vi "Accurate Measure_BU.vi"(0 "DMM ref":refnum<visa-resource-name>, 1 "channel_count":i32=11, 2 "P_current_count":i32, 3 "N_current_count":i32, 5 "DMM error":errorcluster, 7 "Enable DMM-\nRelay":bool=TRUE, 9 "ESP32 ref":refnum<visa-resource-name>, 11 "ESP32 error":errorcluster, 12 "current_mode":u8[](array[numeric])=[0, 0, 0, 0, 0, 0, 0, 0, 0, 0, 0]) -> ()   [LabVIEW 2023]
uses:
  <instrlib>/Agilent 3446X Series/Agilent 3446X Series.lvlib
panel:
  out "time_out_count":i32
  in  "Timeout":i32=100
  out "Arithmetic Mean 3":dbl[](array[numeric])
  out "+ STD":dbl[](array[numeric])
  out "Arithmetic Mean 2":dbl[](array[numeric])
  out "-STD":dbl[](array[numeric])
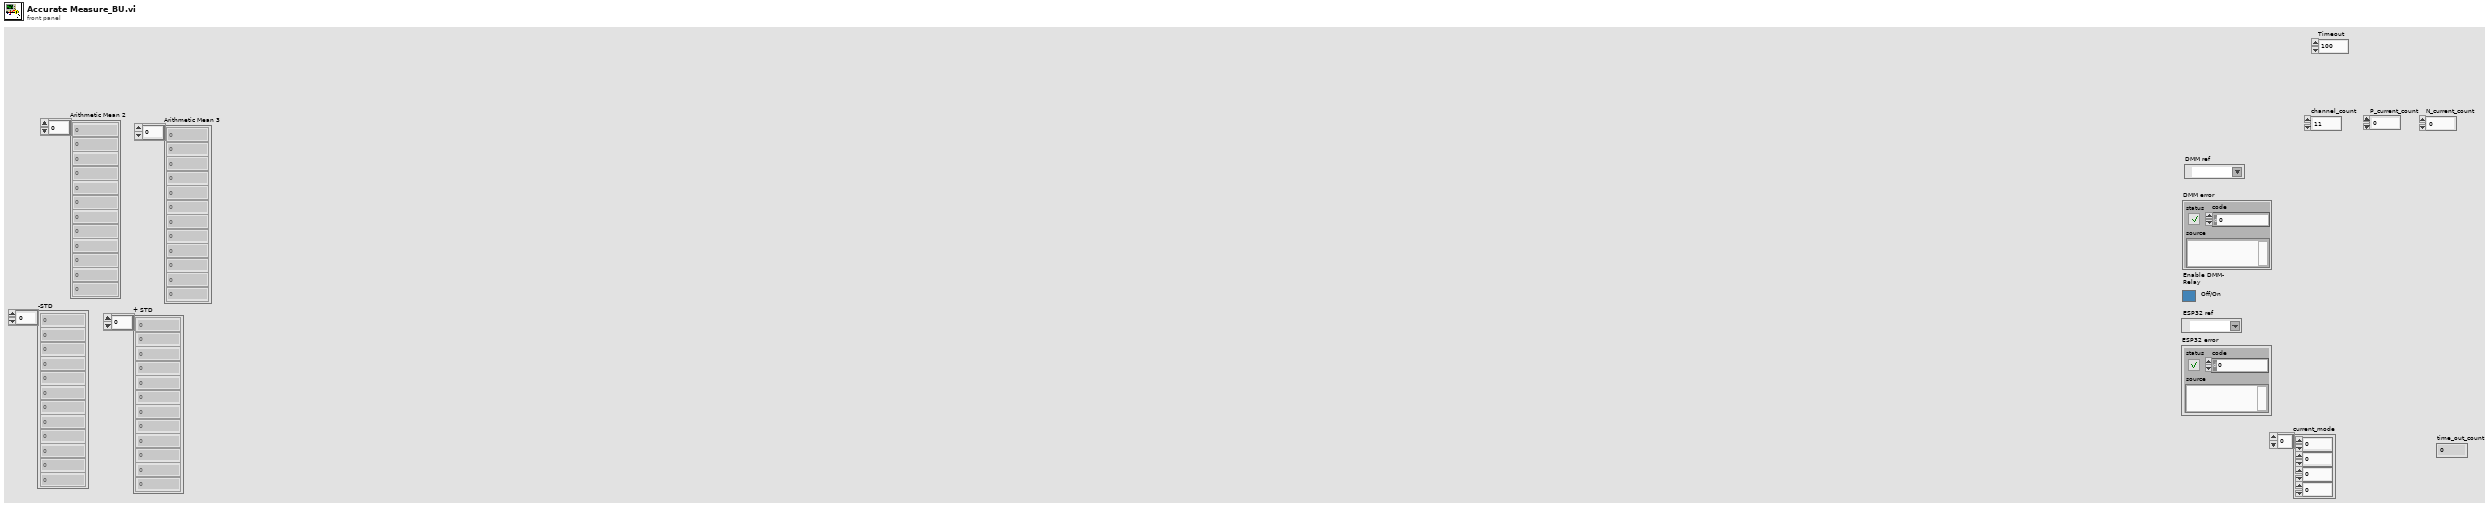
[diagram p1: front panel]
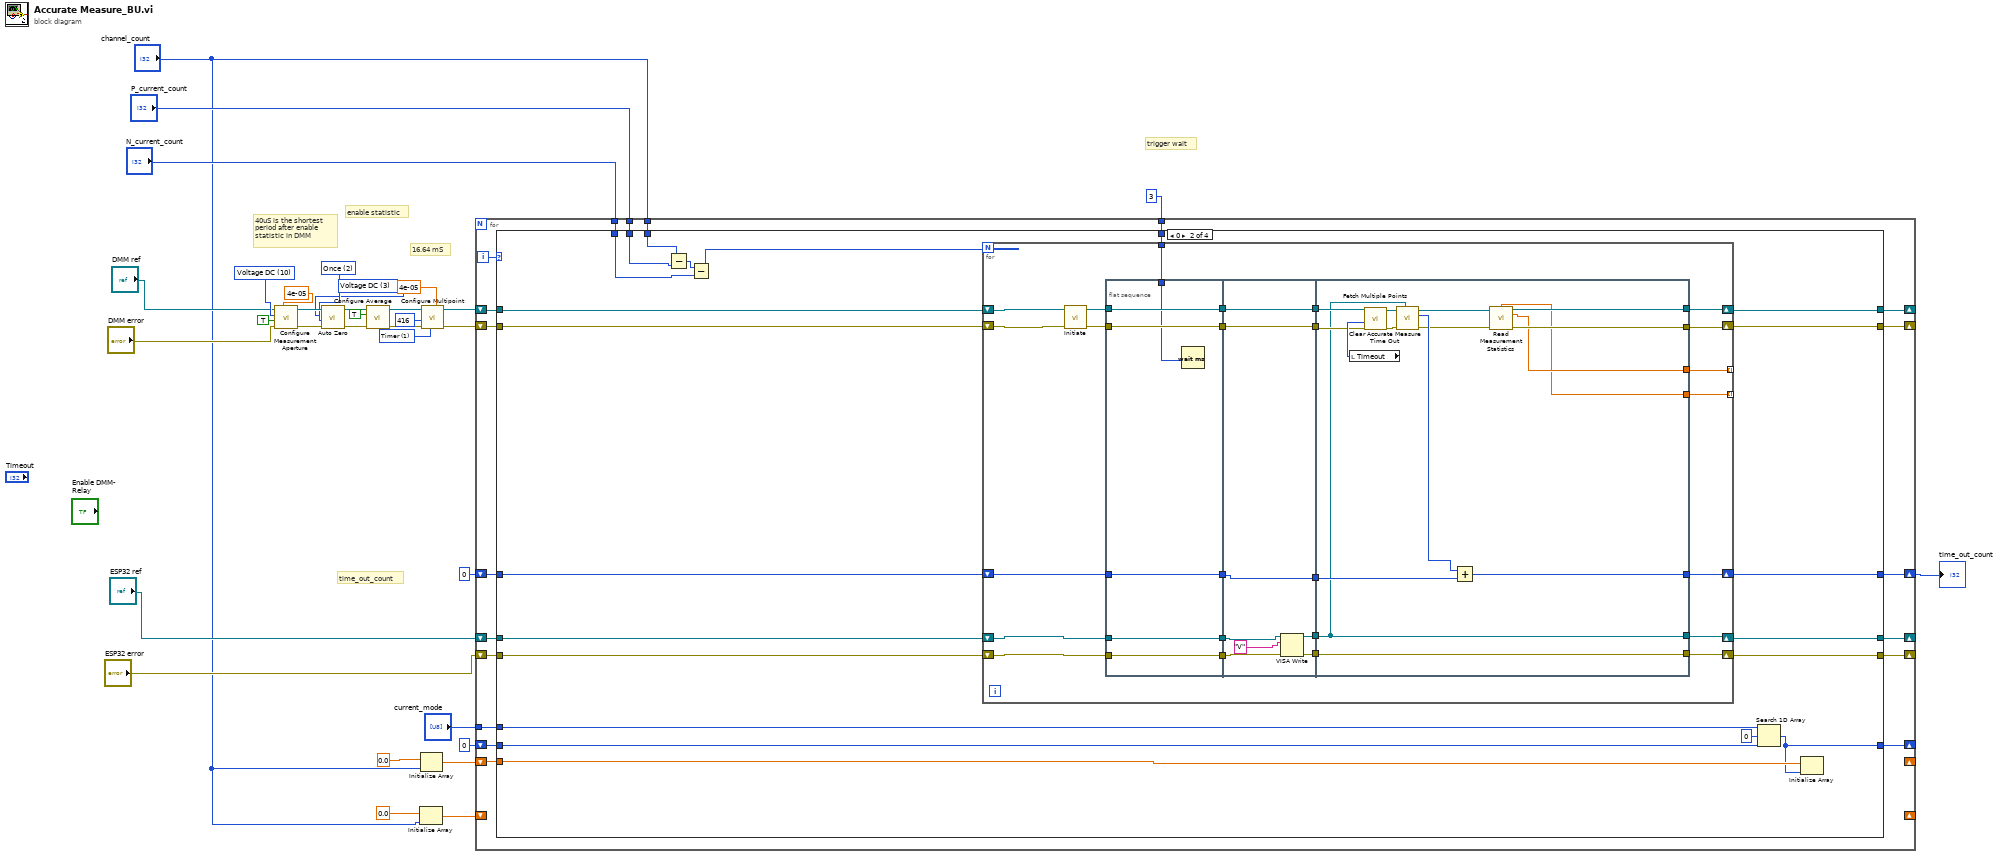
[diagram p0: block diagram]
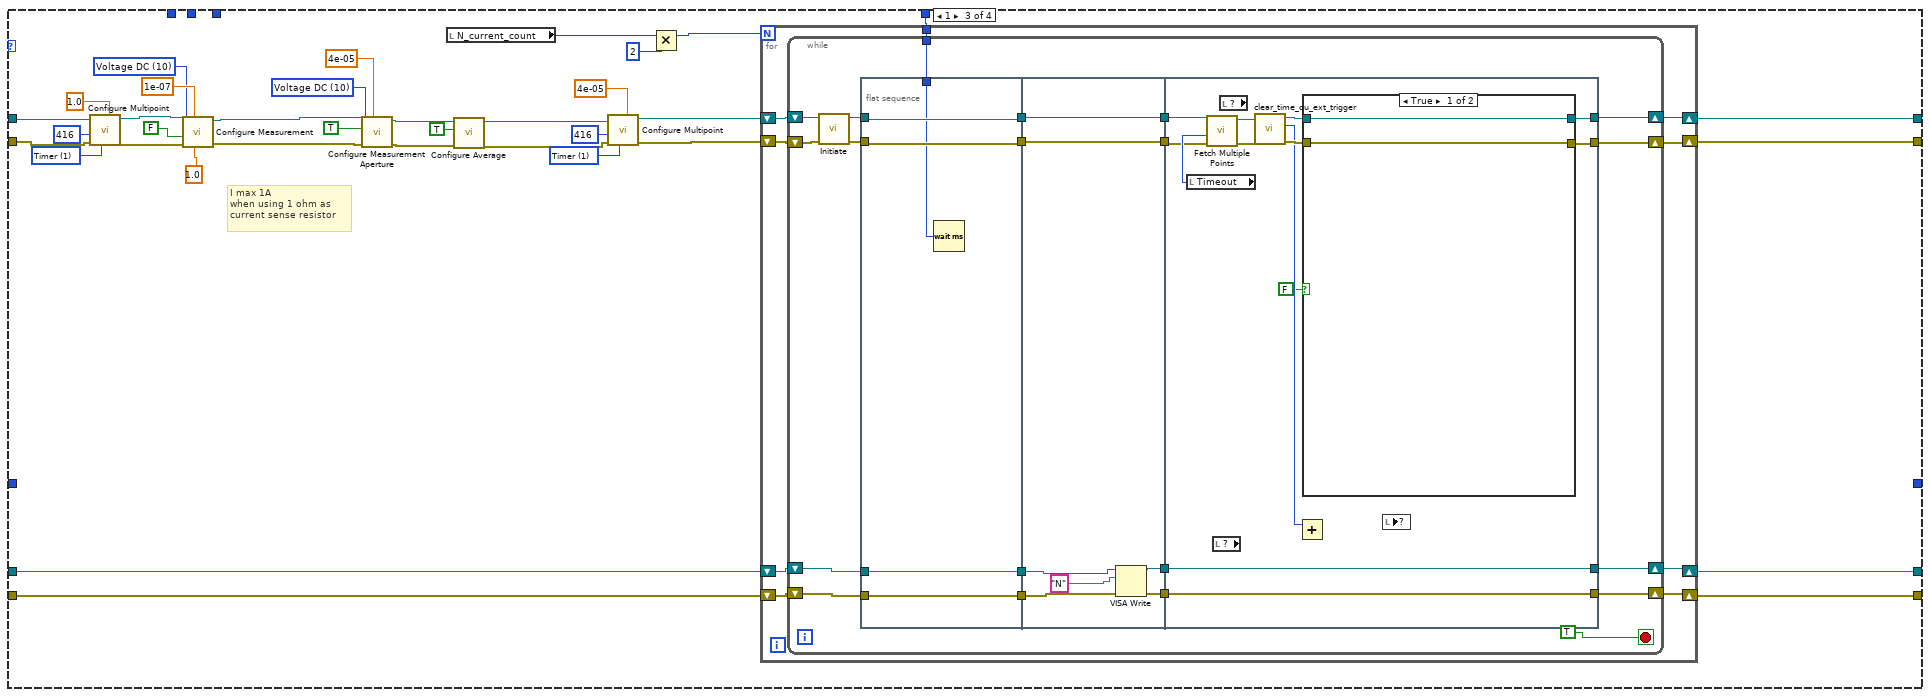
[diagram p3: hidden frame]
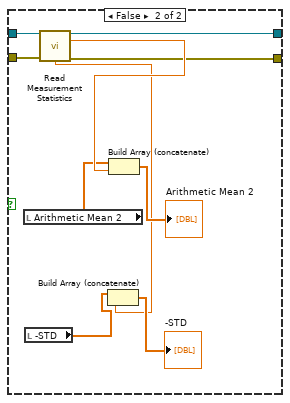
[diagram p4: hidden frame]
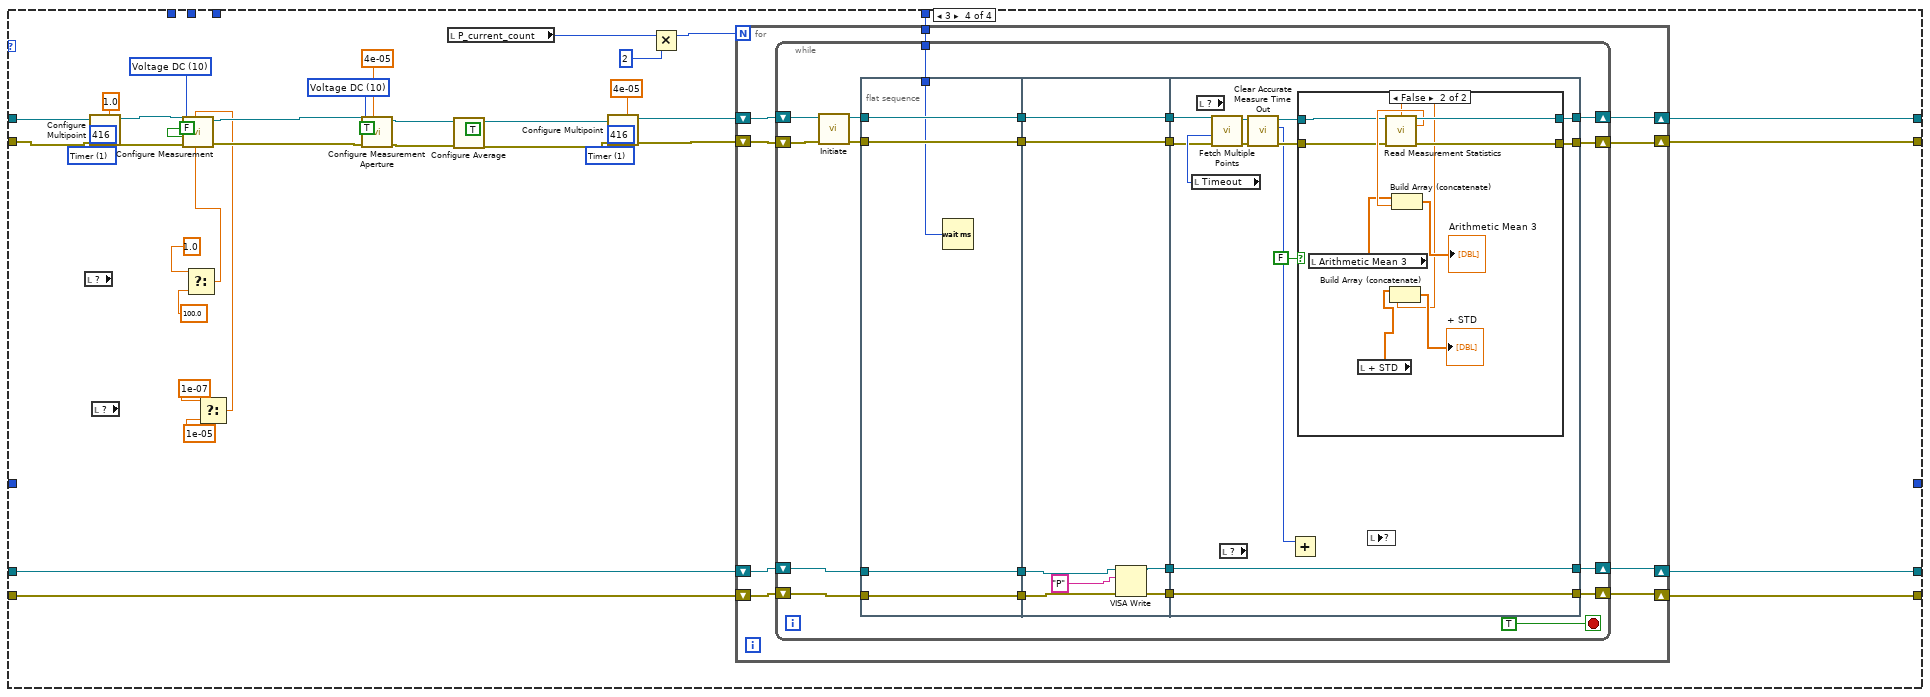
[diagram p5: hidden frame]
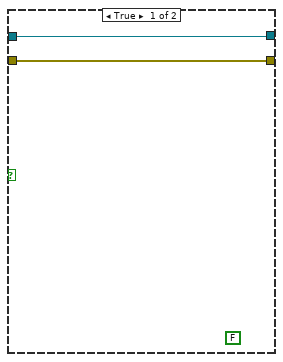
[diagram p6: hidden frame]
diagram:
  w20 = 1 items=["Immediate", "Timer"] ("Sample Source (0: Immediate)")
  w27 = 3 items=["Current DC", "Resistance", "Temperature", "Voltage DC"] ("Zero Type (0: Current DC)")
  w28 = 2 items=["Disable", "Enable", "Once"] ("Auto Zero (1: Enable)")
  w24 = 10 items=["Continuity", "Current AC", "Current DC", "Diode", "Frequency", "Resistance 4-wire", "Period", "Resistance 2-wire", "Temperature", "Voltage AC", "Voltage DC", "Voltage DC Ratio", "Capacitance"] ("Measurement Function (0: Continuity)")
  # "time_out_count"
  # "trigger wait"
  # "16.64 mS"
  # "enable statistic"
  # "40uS is the shortest\nperiod after enable \nstatistic in DMM"
  n1 = call <instrlib>:"Configure Measurement Aperture.vi"("Aperture Time (0.1s)"=4e-05, "error in (no error)"="DMM error", "Enable Aperture (F: Disable)"=TRUE, "Measurement Function (0: Continuity)"=w24, "VISA resource name"="DMM ref") -> ("error out"=w31:errorcluster, "VISA resource name out"=w30:refnum<visa-resource-name>)  [unwired: 5 in]
  n2 = call <instrlib>:"Auto Zero.vi"("error in (no error)"=w31, "Auto Zero (1: Enable)"=w28, "Zero Type (0: Current DC)"=w27, "VISA resource name"=w30) -> ("error out"=w33:errorcluster, "VISA resource name out"=w32:refnum<visa-resource-name>)  [unwired: 6 in]
  n3 = call <instrlib>:"Configure Average.vi"("error in (no error)"=w33, "Enable Statistics (F: Disable)"=TRUE, "VISA resource name"=w32) -> ("error out"=w22:errorcluster, "VISA resource name out"=w23:refnum<visa-resource-name>)  [unwired: 7 in]
  n4 = Initialize Array(0.0 ("Arithmetic Mean"), "channel_count") -> (w2:dbl[])
  n5 = Initialize Array(0.0 ("Arithmetic Mean"), "channel_count") -> (w3:dbl[])
  n6 = call <instrlib>:"Configure Multipoint.vi"("Sample Interval (1 Second)"=4e-05, "Sample Source (0: Immediate)"=w20, "error in (no error)"=w22, "Sample Count (1)"=416, "VISA resource name"=w23) -> ("error out"=w17:errorcluster, "VISA resource name out"=w18:refnum<visa-resource-name>)  [unwired: 2 in, 3 out]
  n7 = for {
    shift-right: [w50] -> _
    shift-left: "ESP32 ref" -> [w52]
    shift-right: [w49] -> _
    shift-left: "ESP32 error" -> [w51]
    shift-right: [w46] -> _
    shift-left: w18 -> [w48]
    shift-right: [w45] -> _
    shift-left: w17 -> [w47]
    tunnel: "channel_count" -> [w44]
    tunnel: "P_current_count" -> [w43]
    tunnel: "N_current_count" -> [w42]
    tunnel: u32 3 ("milliseconds to wait") -> [w41]
    shift-right: [w40] -> w8
    shift-left: 0 -> [w39]
    tunnel: "current_mode" -> [w38]
    shift-right: _ -> [_]
    shift-left: w3 -> [w34]
    shift-right: _ -> [_]
    shift-left: w2 -> [_]
    shift-right: [w36] -> _
    shift-left: 0 ("index of element") -> [w35]
    i -> [w37]
    n8 = case shown="0" w37 {
      tunnel: w52 -> [w54 w73 w168 w274]
      tunnel: w51 -> [w53 w72 w167 w273]
      tunnel: [w54 w69 w164 w270] -> w50
      tunnel: [w53 w68 w163 w269] -> w49
      tunnel: w48 -> [w56 w75 w154 w262]
      tunnel: w47 -> [w55 w74 w153 w261]
      tunnel: [w56 w71 w166 w272] -> w46
      tunnel: [w55 w70 w165 w271] -> w45
      tunnel: w44 -> [_ w67 _ _]
      tunnel: w43 -> [_ w66 _ _]
      tunnel: w42 -> [_ w65 _ _]
      tunnel: [_ w63 _ _] -> w40
      tunnel: w41 -> [_ w64 w133 w235]
      tunnel: w39 -> [_ w62 _ _]
      tunnel: w38 -> [_ w61 _ _]
      tunnel: [_ w57 _ _] -> w36
      tunnel: w35 -> [_ w59 _ _]
      tunnel: w34 -> [_ w58 _ _]
      frame Default {
      }
      frame 0 {
        n9 = Subtract(x=w67, y=w66) -> (x-y=w77:i32)
        n10 = Subtract(x=w77, y=w65) -> (x-y=w76:i32)
        n11 = for {
          N: w76 -> [_]
          shift-right: [w98] -> w71
          shift-left: w75 -> [w102]
          shift-right: [w97] -> w70
          shift-left: w74 -> [w101]
          shift-right: [w96] -> w69
          shift-left: w73 -> [w100]
          shift-right: [w95] -> w68
          shift-left: w72 -> [w99]
          tunnel: w64 -> [w81]
          shift-right: [w80] -> w63
          shift-left: w62 -> [w94]
          tunnel: [w79] -> _ mode=indexing
          tunnel: [w78] -> _ mode=indexing
          n12 = call <instrlib>:"Initiate.vi"("error in (no error)"=w101, "VISA resource name"=w102) -> ("error out"=w82:errorcluster, "VISA resource name out"=w83:refnum<visa-resource-name>)  [unwired: 8 in]
          n13 = flat-sequence {
            tunnel: [w108] -> w93
            tunnel: w100 -> [w108]
            tunnel: [w107] -> w92
            tunnel: w99 -> [w107]
            tunnel: w83 -> [w106]
            tunnel: [w106] -> w91
            tunnel: [w105] -> w90
            tunnel: w82 -> [w105]
            tunnel: [w104] -> w89
            tunnel: w94 -> [w104]
            tunnel: w81 -> [w103]
            tunnel: w93 -> [w116]
            tunnel: w92 -> [w115]
            tunnel: w91 -> [w114]
            tunnel: [w114] -> w85
            tunnel: w90 -> [w113]
            tunnel: [w113] -> w86
            tunnel: [w112] -> w87
            tunnel: [w111] -> w88
            tunnel: w89 -> [w109]
            tunnel: [w109] -> w84
            tunnel: [w132] -> w95
            tunnel: [w119] -> w96
            tunnel: [w123] -> w97
            tunnel: [w124] -> w98
            tunnel: w88 -> [w132]
            tunnel: w87 -> [w119]
            tunnel: w86 -> [w130]
            tunnel: w85 -> [w129]
            tunnel: [w125] -> w80
            tunnel: w84 -> [w120]
            tunnel: [w118] -> w79
            tunnel: [w117] -> w78
            frame #0 {
              n14 = Wait (ms)(milliseconds to wait=w103) -> ()  [unwired: 1 out]
            }
            frame #1 {
              n15 = VISA Write(VISA resource name=w116, write buffer="V" ("data in"), error in (no error)=w115) -> (VISA resource name out=w112:refnum<visa-resource-name>, error out=w111:errorcluster)  [unwired: 1 out]
            }
            frame #2 {
              n16 = local read "Timeout"() -> (w131:i32)
              n17 = call <instrlib>:"Fetch Multiple Points.vi"("error in (no error)"=w130, "Timeout (10000 ms)"=w131, "VISA resource name"=w129) -> ("error out"=w127:errorcluster, "VISA resource name out"=w128:refnum<visa-resource-name>)  [unwired: 1 in, 6 out]
              n18 = call "Clear Accurate Measure Time Out.vi"("ESP32 ref"=w119, "error in (no error)"=w127, "DMM ref"=w128) -> ("error out"=w121:errorcluster, "Time out count"=w126:i32, "VISA Refnum out"=w122:refnum<visa-resource-name>)  [unwired: 5 in, 1 out]
              n19 = Add(x=w126, y=w120) -> (x+y=w125:i32)
              n20 = call <instrlib>:"Read Measurement Statistics.vi"("VISA resource name"=w122, "error in (no error)"=w121) -> ("Standard Deviation"=w117:dbl, "VISA resource name out"=w124:refnum<visa-resource-name>, "Arithmetic Mean"=w118:dbl, "error out"=w123:errorcluster)  [unwired: 6 in, 4 out]
            }
          }
        }
        n21 = Search 1D Array(1D array=w61, element=u8 0, start index (0)=w59) -> (index of element=w57:i32)
        n22 = Initialize Array(w58, w57) -> ()  [unwired: 1 out]
      }
      frame 1 {
        w146 = 1 items=["Immediate", "Timer"] ("Sample Source (0: Immediate)")
        w149 = 10 items=["Continuity", "Current AC", "Current DC", "Diode", "Frequency", "Resistance 4-wire", "Period", "Resistance 2-wire", "Temperature", "Voltage AC", "Voltage DC", "Voltage DC Ratio", "Capacitance"] ("Measurement Function (0: Continuity)")
        w156 = 1 items=["Immediate", "Timer"] ("Sample Source (0: Immediate)")
        w158 = 10 items=["Continuity", "Current AC", "Current DC", "Diode", "Frequency", "Resistance 4-wire", "Period", "Resistance 2-wire", "Temperature", "Voltage AC", "Voltage DC", "Voltage DC Ratio", "Capacitance"] ("Measurement Function (10: Voltage DC)")
        # "I max 1A\nwhen using 1 ohm as \ncurrent sense resistor"
        n23 = call <instrlib>:"Configure Multipoint.vi"("Sample Interval (1 Second)"=1.0, "Sample Source (0: Immediate)"=w156, "error in (no error)"=w153, "Sample Count (1)"=416, "VISA resource name"=w154) -> ("error out"=w138:errorcluster, "VISA resource name out"=w137:refnum<visa-resource-name>)  [unwired: 2 in, 3 out]
        n24 = call <instrlib>:"Configure Measurement.vi"("Manual Range (1)"=1.0, "Absolute Resolution (1E-6)"=1e-07, "error in (no error)"=w138, "Auto Range (T: Enable)"=FALSE, "Measurement Function (10: Voltage DC)"=w158, "VISA resource name"=w137) -> ("error out"=w135:errorcluster, "VISA resource name out"=w136:refnum<visa-resource-name>)  [unwired: 4 out]
        n25 = call <instrlib>:"Configure Measurement Aperture.vi"("Aperture Time (0.1s)"=4e-05, "error in (no error)"=w135, "Enable Aperture (F: Disable)"=TRUE, "Measurement Function (0: Continuity)"=w149, "VISA resource name"=w136) -> ("error out"=w140:errorcluster, "VISA resource name out"=w141:refnum<visa-resource-name>)  [unwired: 5 in]
        n26 = local read "N_current_count"() -> (w162:i32)
        n27 = call <instrlib>:"Configure Average.vi"("error in (no error)"=w140, "Enable Statistics (F: Disable)"=TRUE, "VISA resource name"=w141) -> ("error out"=w139:errorcluster, "VISA resource name out"=w134:refnum<visa-resource-name>)  [unwired: 7 in]
        n28 = call <instrlib>:"Configure Multipoint.vi"("Sample Interval (1 Second)"=4e-05, "Sample Source (0: Immediate)"=w146, "error in (no error)"=w139, "Sample Count (1)"=416, "VISA resource name"=w134) -> ("error out"=w143:errorcluster, "VISA resource name out"=w144:refnum<visa-resource-name>)  [unwired: 2 in, 3 out]
        n29 = Multiply(x=w162, y=2) -> (x*y=w152:i32)
        n30 = for {
          N: w152 -> [_]
          shift-right: [w173] -> w166
          shift-left: w144 -> [w177]
          shift-right: [w172] -> w165
          shift-left: w143 -> [w176]
          shift-right: [w171] -> w164
          shift-left: w168 -> [w175]
          shift-right: [w170] -> w163
          shift-left: w167 -> [w174]
          tunnel: w133 -> [w169]
          n31 = while {
            shift-right: [w183] -> w173
            shift-left: w177 -> [w189]
            shift-right: [w182] -> w172
            shift-left: w176 -> [w188]
            shift-right: [w181] -> w171
            shift-left: w175 -> [w187]
            shift-right: [w180] -> w170
            shift-left: w174 -> [w186]
            tunnel: w169 -> [w178]
            stop <- TRUE stop-if-true
            n32 = call <instrlib>:"Initiate.vi"("error in (no error)"=w188, "VISA resource name"=w189) -> ("error out"=w184:errorcluster, "VISA resource name out"=w185:refnum<visa-resource-name>)  [unwired: 8 in]
            n33 = flat-sequence {
              tunnel: [w202] -> w197
              tunnel: w187 -> [w202]
              tunnel: [w201] -> w196
              tunnel: w186 -> [w201]
              tunnel: w185 -> [w200]
              tunnel: [w200] -> w195
              tunnel: [w199] -> w194
              tunnel: w184 -> [w199]
              tunnel: w178 -> [w198]
              tunnel: w197 -> [w209]
              tunnel: w196 -> [w208]
              tunnel: w195 -> [w207]
              tunnel: [w207] -> w193
              tunnel: w194 -> [w206]
              tunnel: [w206] -> w192
              tunnel: [w205] -> w191
              tunnel: [w204] -> w190
              tunnel: w193 -> [w218]
              tunnel: w192 -> [w219]
              tunnel: [w213] -> w183
              tunnel: [w212] -> w182
              tunnel: [w222] -> w181
              tunnel: w191 -> [w222]
              tunnel: [w221] -> w180
              tunnel: w190 -> [w221]
              frame #0 {
                n34 = Wait (ms)(milliseconds to wait=w198) -> ()  [unwired: 1 out]
              }
              frame #1 {
                n35 = VISA Write(VISA resource name=w209, write buffer="N" ("data in"), error in (no error)=w208) -> (VISA resource name out=w205:refnum<visa-resource-name>, error out=w204:errorcluster)  [unwired: 1 out]
              }
              frame #2 {
                n36 = local read "Timeout"() -> (w220:i32)
                n37 = call <instrlib>:"Fetch Multiple Points.vi"("error in (no error)"=w219, "Timeout (10000 ms)"=w220, "VISA resource name"=w218) -> ("error out"=w216:errorcluster, "VISA resource name out"=w217:refnum<visa-resource-name>)  [unwired: 1 in, 6 out]
                n38 = local read item#-1() -> ()  [unwired: 1 out]
                n39 = local read item#-1() -> ()  [unwired: 1 out]
                n40 = call "clear_time_ou_ext_trigger.vi"("error in (no error)"=w216, "VISA Refnum in"=w217) -> ("error out"=w214:errorcluster, "Time out count"=w211:i32, "VISA Refnum out"=w215:refnum<visa-resource-name>)  [unwired: 6 in, 1 out]
                n41 = Add(x=w211) -> ()  [unwired: 1 in, 1 out]
                n42 = case shown="True" FALSE {
                  tunnel: w215 -> [w224 w228]
                  tunnel: w214 -> [w223 w227]
                  tunnel: [w224 w226] -> w213
                  tunnel: [w223 w225] -> w212
                  frame True {
                  }
                  frame False {
                    n43 = local read "Arithmetic Mean 2"() -> (w233:dbl[])
                    n44 = local read "-STD"() -> (w231:dbl[])
                    n45 = call <instrlib>:"Read Measurement Statistics.vi"("VISA resource name"=w228, "error in (no error)"=w227) -> ("Standard Deviation"=w229:dbl, "VISA resource name out"=w226:refnum<visa-resource-name>, "Arithmetic Mean"=w234:dbl, "error out"=w225:errorcluster)  [unwired: 6 in, 4 out]
                    n46 = Build Array (concatenate)(w231, w229) -> (→"-STD":dbl[])
                    n47 = Build Array (concatenate)(w233, w234) -> (→"Arithmetic Mean 2":dbl[])
                  }
                }
                n48 = local read item#-1() -> ()  [unwired: 1 in]
              }
            }
          }
        }
      }
      frame 3 {
        w254 = 1 items=["Immediate", "Timer"] ("Sample Source (0: Immediate)")
        w257 = 10 items=["Continuity", "Current AC", "Current DC", "Diode", "Frequency", "Resistance 4-wire", "Period", "Resistance 2-wire", "Temperature", "Voltage AC", "Voltage DC", "Voltage DC Ratio", "Capacitance"] ("Measurement Function (0: Continuity)")
        w264 = 1 items=["Immediate", "Timer"] ("Sample Source (0: Immediate)")
        w266 = 10 items=["Continuity", "Current AC", "Current DC", "Diode", "Frequency", "Resistance 4-wire", "Period", "Resistance 2-wire", "Temperature", "Voltage AC", "Voltage DC", "Voltage DC Ratio", "Capacitance"] ("Measurement Function (10: Voltage DC)")
        n49 = local read item#-1() -> ()  [unwired: 1 out]
        n50 = call <instrlib>:"Configure Multipoint.vi"("Sample Interval (1 Second)"=1.0, "Sample Source (0: Immediate)"=w264, "error in (no error)"=w261, "Sample Count (1)"=416, "VISA resource name"=w262) -> ("error out"=w246:errorcluster, "VISA resource name out"=w245:refnum<visa-resource-name>)  [unwired: 2 in, 3 out]
        n51 = local read item#-1() -> ()  [unwired: 1 out]
        n52 = Select(t=1.0 ("Manual Range (1)"), f=100.0 ("Manual Range (1)")) -> (s? t:f=w239:dbl)  [unwired: 1 in]
        n53 = Select(t=1e-07 ("Absolute Resolution (1E-6)"), f=1e-05 ("Absolute Resolution (1E-6)")) -> (s? t:f=w236:dbl)  [unwired: 1 in]
        n54 = call <instrlib>:"Configure Measurement.vi"("Manual Range (1)"=w239, "Absolute Resolution (1E-6)"=w236, "error in (no error)"=w246, "Auto Range (T: Enable)"=FALSE, "Measurement Function (10: Voltage DC)"=w266, "VISA resource name"=w245) -> ("error out"=w243:errorcluster, "VISA resource name out"=w244:refnum<visa-resource-name>)  [unwired: 4 out]
        n55 = call <instrlib>:"Configure Measurement Aperture.vi"("Aperture Time (0.1s)"=4e-05, "error in (no error)"=w243, "Enable Aperture (F: Disable)"=TRUE, "Measurement Function (0: Continuity)"=w257, "VISA resource name"=w244) -> ("error out"=w248:errorcluster, "VISA resource name out"=w249:refnum<visa-resource-name>)  [unwired: 5 in]
        n56 = local read "P_current_count"() -> (w268:i32)
        n57 = call <instrlib>:"Configure Average.vi"("error in (no error)"=w248, "Enable Statistics (F: Disable)"=TRUE, "VISA resource name"=w249) -> ("error out"=w247:errorcluster, "VISA resource name out"=w242:refnum<visa-resource-name>)  [unwired: 7 in]
        n58 = call <instrlib>:"Configure Multipoint.vi"("Sample Interval (1 Second)"=4e-05, "Sample Source (0: Immediate)"=w254, "error in (no error)"=w247, "Sample Count (1)"=416, "VISA resource name"=w242) -> ("error out"=w251:errorcluster, "VISA resource name out"=w252:refnum<visa-resource-name>)  [unwired: 2 in, 3 out]
        n59 = Multiply(x=w268, y=2) -> (x*y=w260:i32)
        n60 = for {
          N: w260 -> [_]
          shift-right: [w279] -> w272
          shift-left: w252 -> [w283]
          shift-right: [w278] -> w271
          shift-left: w251 -> [w282]
          shift-right: [w277] -> w270
          shift-left: w274 -> [w281]
          shift-right: [w276] -> w269
          shift-left: w273 -> [w280]
          tunnel: w235 -> [w275]
          n61 = while {
            shift-right: [w289] -> w279
            shift-left: w283 -> [w295]
            shift-right: [w288] -> w278
            shift-left: w282 -> [w294]
            shift-right: [w287] -> w277
            shift-left: w281 -> [w293]
            shift-right: [w286] -> w276
            shift-left: w280 -> [w292]
            tunnel: w275 -> [w284]
            stop <- TRUE stop-if-true
            n62 = call <instrlib>:"Initiate.vi"("error in (no error)"=w294, "VISA resource name"=w295) -> ("error out"=w290:errorcluster, "VISA resource name out"=w291:refnum<visa-resource-name>)  [unwired: 8 in]
            n63 = flat-sequence {
              tunnel: [w308] -> w303
              tunnel: w293 -> [w308]
              tunnel: [w307] -> w302
              tunnel: w292 -> [w307]
              tunnel: w291 -> [w306]
              tunnel: [w306] -> w301
              tunnel: [w305] -> w300
              tunnel: w290 -> [w305]
              tunnel: w284 -> [w304]
              tunnel: w303 -> [w315]
              tunnel: w302 -> [w314]
              tunnel: w301 -> [w313]
              tunnel: [w313] -> w299
              tunnel: w300 -> [w312]
              tunnel: [w312] -> w298
              tunnel: [w311] -> w297
              tunnel: [w310] -> w296
              tunnel: w299 -> [w322]
              tunnel: w298 -> [w323]
              tunnel: [w328] -> w289
              tunnel: [w327] -> w288
              tunnel: [w326] -> w287
              tunnel: w297 -> [w326]
              tunnel: [w325] -> w286
              tunnel: w296 -> [w325]
              frame #0 {
                n64 = Wait (ms)(milliseconds to wait=w304) -> ()  [unwired: 1 out]
              }
              frame #1 {
                n65 = VISA Write(VISA resource name=w315, write buffer="P" ("data in"), error in (no error)=w314) -> (VISA resource name out=w311:refnum<visa-resource-name>, error out=w310:errorcluster)  [unwired: 1 out]
              }
              frame #2 {
                n66 = local read "Timeout"() -> (w324:i32)
                n67 = local read item#-1() -> ()  [unwired: 1 out]
                n68 = call <instrlib>:"Fetch Multiple Points.vi"("error in (no error)"=w323, "Timeout (10000 ms)"=w324, "VISA resource name"=w322) -> ("error out"=w320:errorcluster, "VISA resource name out"=w321:refnum<visa-resource-name>)  [unwired: 1 in, 6 out]
                n69 = local read item#-1() -> ()  [unwired: 1 out]
                n70 = call "Clear Accurate Measure Time Out.vi"("error in (no error)"=w320, "DMM ref"=w321) -> ("error out"=w318:errorcluster, "Time out count"=w317:i32, "VISA Refnum out"=w319:refnum<visa-resource-name>)  [unwired: 6 in, 1 out]
                n71 = Add(x=w317) -> ()  [unwired: 1 in, 1 out]
                n72 = case shown="False" FALSE {
                  tunnel: [w330 w340] -> w328
                  tunnel: [w329 w339] -> w327
                  tunnel: w319 -> [w330 w337]
                  tunnel: w318 -> [w329 w336]
                  frame True {
                    (unwired) FALSE
                  }
                  frame False {
                    n73 = local read "Arithmetic Mean 3"() -> (w335:dbl[])
                    n74 = local read "+ STD"() -> (w333:dbl[])
                    n75 = call <instrlib>:"Read Measurement Statistics.vi"("VISA resource name"=w337, "error in (no error)"=w336) -> ("Standard Deviation"=w331:dbl, "VISA resource name out"=w340:refnum<visa-resource-name>, "Arithmetic Mean"=w338:dbl, "error out"=w339:errorcluster)  [unwired: 6 in, 4 out]
                    n76 = Build Array (concatenate)(w333, w331) -> (→"+ STD":dbl[])
                    n77 = Build Array (concatenate)(w335, w338) -> (→"Arithmetic Mean 3":dbl[])
                  }
                }
                n78 = local read item#-1() -> ()  [unwired: 1 in]
              }
            }
          }
        }
      }
    }
  }
  "time_out_count" <- w8
